vi "EminemCmdIntake.vi"(8 "error in (no error)":errorcluster, 11 "Box intake":bool) -> (0 "error out":errorcluster)   [LabVIEW 2023]
uses:
  <vilib>/Rock Robotics/WPI/ThirdParty/JAS_Junk/TrajLib/Trajectory_Library.lvlib
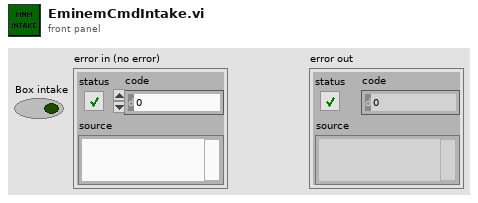
[diagram p1: front panel]
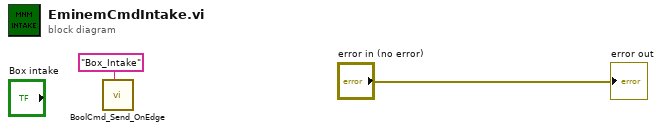
[diagram p0: block diagram]
diagram:
  n1 = call <vilib>:"BoolCmd_Send_OnEdge.vi"("Command Name"="Box_Intake") -> ()  [unwired: 10 in, 1 out]
  "error out" <- "error in (no error)"
